vi "WhileLoopIter.vi"() -> ()   [LabVIEW 2019]
panel:
  out "IteratorValue":i32
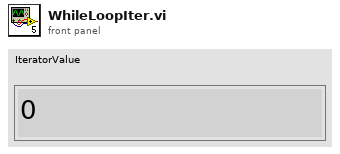
[diagram p1: front panel]
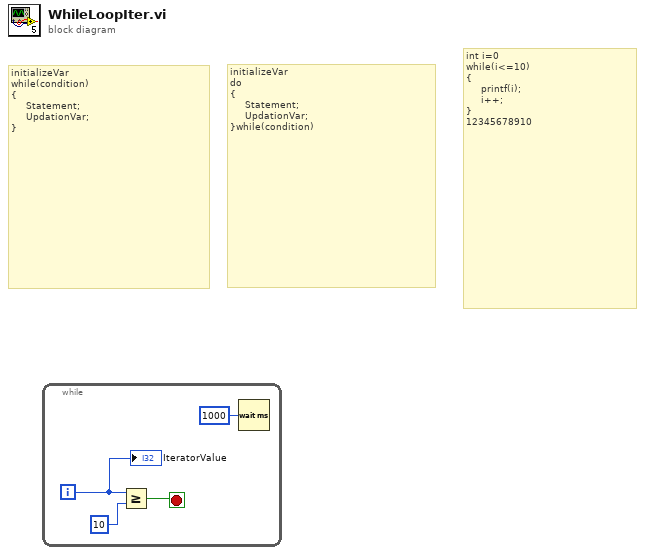
[diagram p0: block diagram]
diagram:
  # "int i=0\nwhile(i<=10)\n{\n     printf(i);\n     i++;\n}\n12345678910"
  # "initializeVar\ndo\n{\n     Statement;\n     UpdationVar;\n}while(condition)"
  # "initializeVar\nwhile(condition)\n{\n     Statement;\n     UpdationVar;\n}"
  n1 = while {
    i -> [w4]
    stop <- w2 stop-if-true
    n2 = Greater Or Equal?(x=w4, y=10) -> (x >= y?=w2:bool)
    n3 = Wait (ms)(milliseconds to wait=u32 1000) -> ()  [unwired: 1 out]
    "IteratorValue" <- w4
  }
